vi "Get Channel Timing.vi"(8 "dt":dbl, 9 "T0":timestamp, 10 "Resample":bool, 11 "Time Format":string) -> (3 "Channel Stats":string[](array[string]))   [LabVIEW 2022 SP3, in "CSV Export.lvlib" / "CSV Export.lvclass"]
uses:
  CSV Export.lvclass
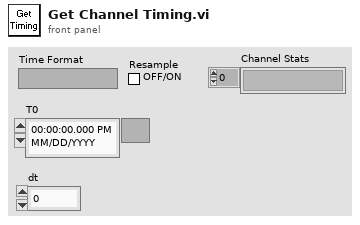
[diagram p1: front panel]
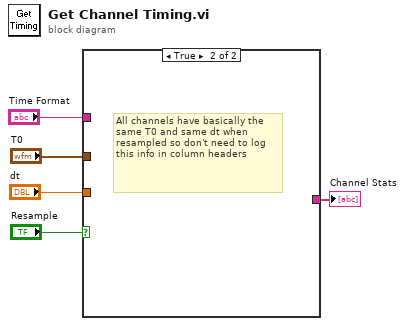
[diagram p0: block diagram]
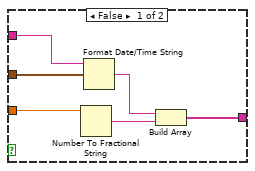
[diagram p2: hidden frame]
diagram:
  n1 = case shown="True" "Resample" {
    tunnel: [w10 _] -> w4
    tunnel: "dt" -> [w9 _]
    tunnel: "T0" -> [w8 _]
    tunnel: "Time Format" -> [w7 _]
    frame False {
      n2 = Number To Fractional String(number=w9) -> (F-format string=w11:string)  [unwired: 3 in]
      n3 = Format Date/Time String(time format string (%c)=w7, seconds (now)=w8) -> (date/time string=w6:string)  [unwired: 1 in]
      n4 = Build Array(w6, w11) -> (w10:string[])
    }
    frame True {
      # "All channels have basically the same T0 and same dt when resampled so don't need to log this info in column headers"
    }
  }
  "Channel Stats" <- w4
